vi "slopes2zern.vi"(0 "HasoSlopes in":refnum<class "HasoSlopes.lvclass">, 3 "error in (no error)":errorcluster, 4 "idxType":enum16{"Wyant", "ANSI"}(ring)) -> (6 "HasoSlopes out":refnum<class "HasoSlopes.lvclass">, 7 "Zernike Coefficients":dbl[](graph), 8 "Measured pupil":i32[][](graph), 9 "Zernike pupil":i32[][](graph), 10 "error out":errorcluster)   [LabVIEW 2018]
uses:
  <userlib>/WaveKit.lib/Controls/HasoSlopes.lvclass
  <userlib>/WaveKit.lib/Classes/ComputePhaseSet/ComputePhaseSet.lvclass
  <userlib>/WaveKit.lib/Controls/Pupil.lvclass
  <userlib>/WaveKit.lib/Controls/CircularPupilDetectionParams.ctl
  <userlib>/WaveKit.lib/Controls/PupilDetectionOption.ctl
  <userlib>/WaveKit.lib/Controls/CircularAutoDetectionOptions.ctl
  <userlib>/WaveKit.lib/Controls/PupilDetectionMode.ctl
  <userlib>/WaveKit.lib/Controls/ZernikeModalPrefs.ctl
  <userlib>/WaveKit.lib/Controls/ZernikeProjectionPupilSetup.ctl
  <userlib>/WaveKit.lib/Controls/Point2Df.ctl
  <userlib>/WaveKit.lib/Classes/ModalCoef/ModalCoef.lvclass
  <userlib>/WaveKit.lib/Controls/WavefrontReconstructionMode.ctl
  <userlib>/WaveKit.lib/Controls/WavefrontModalReconstructionType.ctl
  <userlib>/WaveKit.lib/Classes/HasoData/HasoData.lvclass
  <vilib>/Analysis/1siggen.llb/Ramp Pattern by Delta.vi
  <vilib>/Analysis/NI_AALBase.lvlib
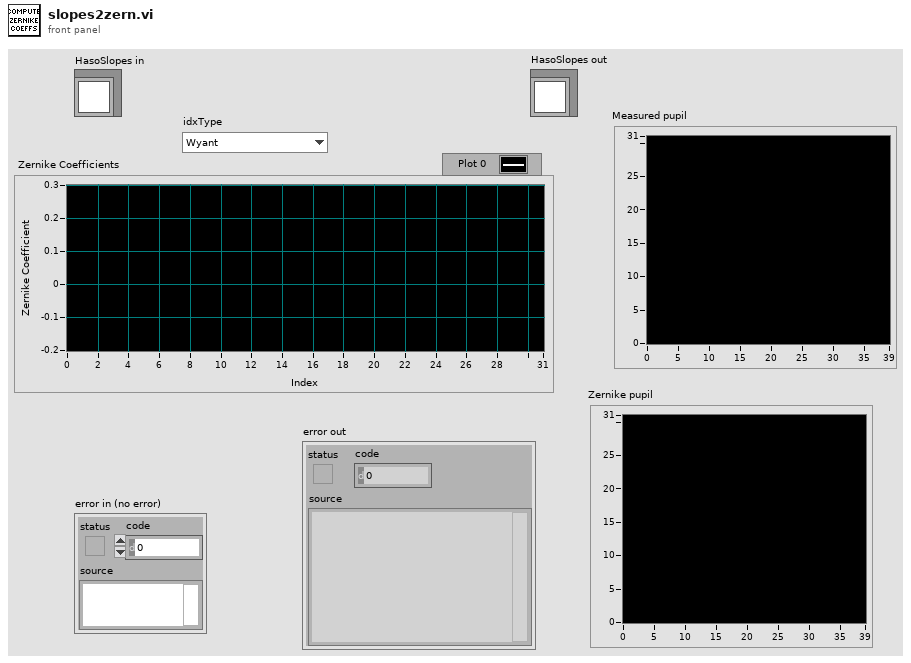
[diagram p1: front panel]
types:
  T1 = typedef "WavefrontModalReconstructionType.ctl" = enum16{"Legendre", "Zernike"}
  T2 = typedef "WavefrontReconstructionMode.ctl" = enum16{"None", "Modal_Legendre", "Modal_Zernike", "Zonal", "Modal_Zonal_Zernike", "Modal_Zonal_Legendre"}
  T3 = typedef "ZernikeModalPrefs.ctl" = cluster{"Number of coefficients":u32, "Filtered coefficients":u32[], "RMS Zernike normalization":bool, "CircularProjectionPupilDimensions":T4}
  T4 = typedef "ZernikeProjectionPupilSetup.ctl" = cluster{"Pupil center_sspp":T5, "Pupil radius_sspp":sgl}
  T5 = typedef "Point2Df.ctl" = cluster{"X":sgl, "Y":sgl}
  T6 = typedef "CircularPupilDetectionParams.ctl" = cluster{"PupilDetectionOption":T7, "AutoDetectionOption":T8, "PupilDetectionMode":T9, "CentralOccultationDetection":bool}
  T7 = typedef "PupilDetectionOption.ctl" = enum16{"Manual", "Automatic"}
  T8 = typedef "CircularAutoDetectionOptions.ctl" = enum16{"manual_radius_auto_center", "manual_center_auto_radius", "auto_radius_auto_center"}
  T9 = typedef "PupilDetectionMode.ctl" = enum16{"inscribed", "circumscribed"}
  T10 = enum16{"ANSI2Wyant", "Wyant2ANSI", "ANSI2ANSI", "Wyant2Wyant"}
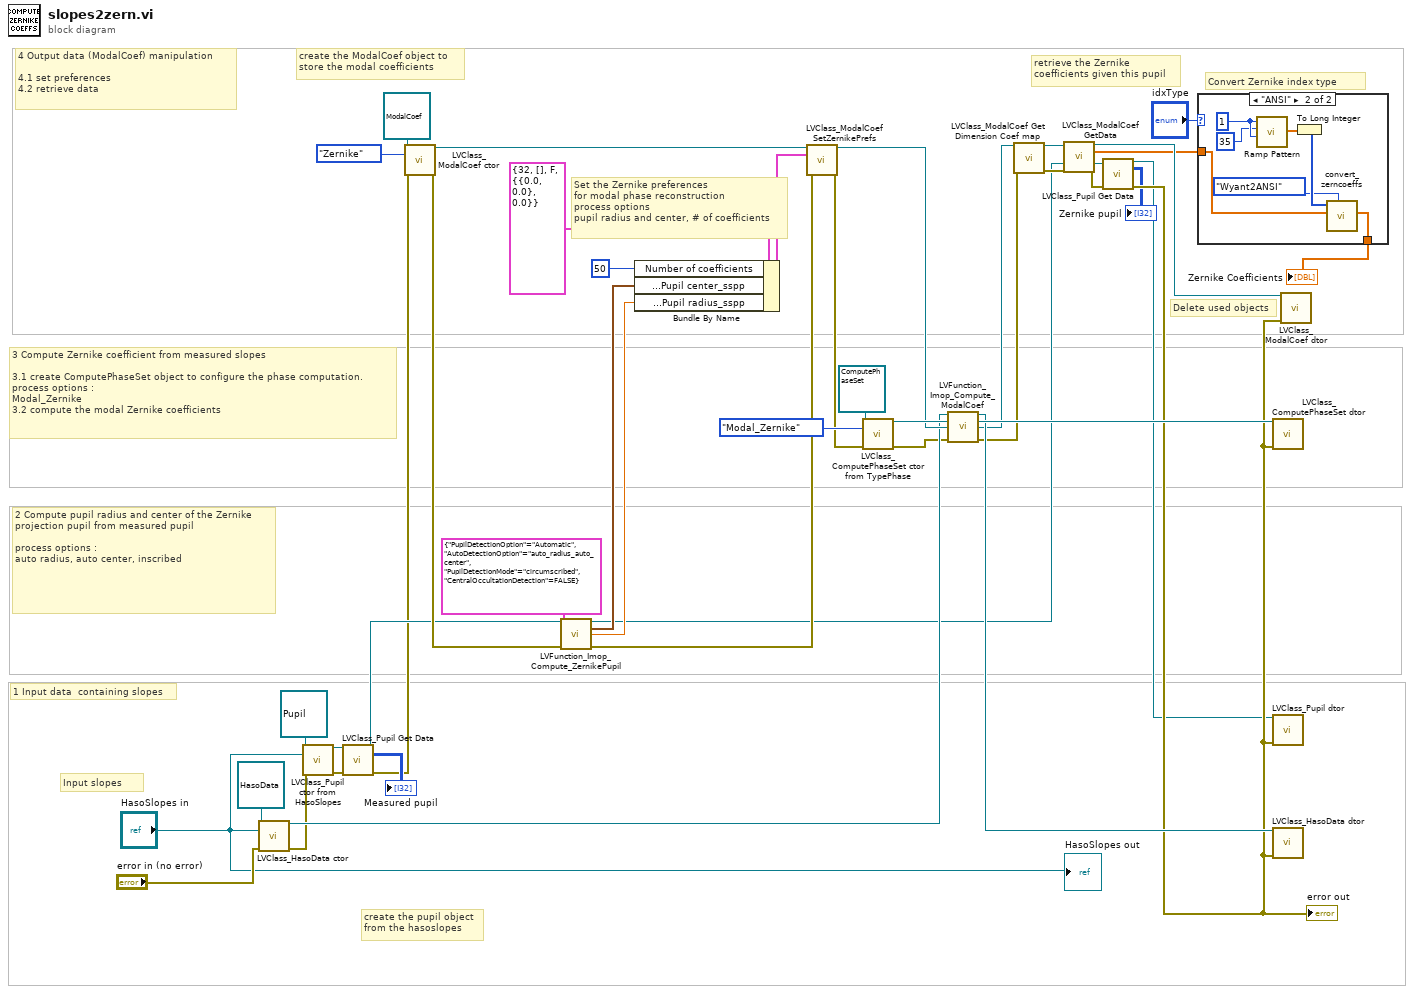
[diagram p0: block diagram]
diagram:
  # "Convert Zernike index type"
  # "Input slopes"
  # "Delete used objects"
  # "4 Output data (ModalCoef) manipulation\n\n4.1 set preferences\n4.2 retrieve data"
  # "retrieve the Zernike\ncoefficients given this pupil"
  # "create the ModalCoef object to\nstore the modal coefficients"
  # "3 Compute Zernike coefficient from measured slopes\n\n3.1 create ComputePhaseSet object to configure the phase computation.\nprocess options :\nModal_Zernike\n3.2 compute the modal Zernike coefficients"
  # "2 Compute pupil radius and center of the Zernike\nprojection pupil from measured pupil\n\nprocess options :\nauto radius, auto center, inscribed"
  # "1 Input data  containing slopes"
  # "Set the Zernike preferences\nfor modal phase reconstruction\nprocess options\npupil radius and center, # of coefficients"
  # "create the pupil object\nfrom the hasoslopes"
  n1 = call <userlib>:"LVClass_HasoData ctor.vi"("HasoData in"=refnum<class "HasoData.lvclass"> refnum, "HasoSlopes.lvclass"="HasoSlopes in", "error in (no error)"="error in (no error)") -> ("HasoData out"=w24:refnum<class "HasoData.lvclass">, "error out"=w22:errorcluster)  [unwired: 11 in]
  n2 = call <userlib>:"LVClass_Pupil ctor from HasoSlopes.vi"("Pupil in"=refnum<class "Pupil.lvclass"> refnum, "HasoSlopes.lvclass"="HasoSlopes in", "error in (no error)"=w22) -> ("Pupil out"=w20:refnum<class "Pupil.lvclass">, "error out"=w18:errorcluster)  [unwired: 11 in]
  n3 = call <userlib>:"LVClass_Pupil Get Data.vi"("Pupil in"=w20, "error in (no error)"=w18) -> ("Pupil out"=w19:refnum<class "Pupil.lvclass">, "Data"=→"Measured pupil":i32[][], "error out"=w8:errorcluster)  [unwired: 11 in]
  n4 = call <userlib>:"LVClass_ModalCoef ctor.vi"("ModalCoef in"=refnum<class "ModalCoef.lvclass"> refnum, "TypePhase"=WavefrontModalReconstructionType."Zernike", "error in (no error)"=w8) -> ("ModalCoef out"=w26:refnum<class "ModalCoef.lvclass">, "error out"=w21:errorcluster)  [unwired: 11 in]
  n5 = call <userlib>:"LVFunction_Imop_Compute_ZernikePupil.vi"("Pupil.lvclass"=w19, "CircularPupilDetectionParams"=T6 {"PupilDetectionOption"=enum."Automatic", "AutoDetectionOption"=enum."auto_radius_auto_center", "PupilDetectionMode"=enum."circumscribed", "CentralOccultationDetection"=FALSE}, "error in"=w21) -> ("Pupil.lvclass"=w15:refnum<class "Pupil.lvclass">, "center"=w32:T5, "radius"=w31:sgl, "error out"=w16:errorcluster)  [unwired: 9 in]
  n6 = Bundle By Name(cluster=T3 {"Number of coefficients"=32, "Filtered coefficients"=[], "RMS Zernike normalization"=FALSE, "CircularProjectionPupilDimensions"={"Pupil center_sspp"={"X"=0.0, "Y"=0.0}, "Pupil radius_sspp"=0.0}} ("ZernikeModalPrefs"), "Number of coefficients"=u32 50, "CircularProjectionPupilDimensions.Pupil center_sspp"=w32, "CircularProjectionPupilDimensions.Pupil radius_sspp"=w31) -> (w33:T3)
  n7 = call <userlib>:"LVClass_ModalCoef SetZernikePrefs.vi"("ModalCoef in"=w26, "ZernikeModalPrefs"=w33, "error in (no error)"=w16) -> ("ModalCoef out"=w27:refnum<class "ModalCoef.lvclass">, "error out"=w7:errorcluster)  [unwired: 11 in]
  n8 = call <userlib>:"LVClass_ComputePhaseSet ctor from TypePhase.vi"("ComputePhaseSet in"=refnum<class "ComputePhaseSet.lvclass"> refnum, "TypePhase"=WavefrontReconstructionMode."Modal_Zernike", "error in (no error)"=w7) -> ("ComputePhaseSet out"=w28:refnum<class "ComputePhaseSet.lvclass">, "error out"=w6:errorcluster)  [unwired: 11 in]
  n9 = call <userlib>:"LVFunction_Imop_Compute_ModalCoef.vi"("HasoData.lvclass"=w24, "ComputePhaseSet.lvclass"=w28, "ModalCoef.lvclass"=w27, "error constant"=w6) -> ("HasoData.lvclass (dup)"=w38:refnum<class "HasoData.lvclass">, "ComputePhaseSet.lvclass (dup)"=w39:refnum<class "ComputePhaseSet.lvclass">, "ModalCoef.lvclass (dup)"=w23:refnum<class "ModalCoef.lvclass">, "error out"=w35:errorcluster)  [unwired: 8 in]
  n10 = call <userlib>:"LVClass_ModalCoef Get Dimension Coef map.vi"("ModalCoef in"=w23, "error in (no error)"=w35) -> ("ModalCoef out"=w40:refnum<class "ModalCoef.lvclass">, "error out"=w36:errorcluster)  [unwired: 11 in, 1 out]
  n11 = call <userlib>:"LVClass_ModalCoef GetData.vi"("ModalCoef in"=w40, "Pupil.lvclass"=w15, "error in (no error)"=w36) -> ("ModalCoef out"=w37:refnum<class "ModalCoef.lvclass">, "coef"=w2:sgl[], "Pupil.lvclass (dup)"=w13:refnum<class "Pupil.lvclass">, "error out"=w12:errorcluster)  [unwired: 8 in, 1 out]
  n12 = call <userlib>:"LVClass_Pupil Get Data.vi"("Pupil in"=w13, "error in (no error)"=w12) -> ("Pupil out"=w10:refnum<class "Pupil.lvclass">, "Data"=→"Zernike pupil":i32[][], "error out"=w11:errorcluster)  [unwired: 11 in]
  "error out" <- w11
  n13 = case shown="\"ANSI\"" "idxType" {
    tunnel: w2 -> [w45 w51]
    tunnel: [w45 w52] -> w1
    frame "Wyant", Default {
    }
    frame "ANSI" {
      w49 = 1
      n14 = call-poly <vilib>:"Ramp Pattern.vi"("start"=w49, "end"=35, "delta"=w49) -> ("Ramp Pattern"=w50:dbl[])  [unwired: 6 in, 2 out]
      n15 = To Long Integer(number=w50) -> (32bit integer=w47:i32[])
      n16 = call "convert_zerncoeffs.vi"("ConType"=T10."Wyant2ANSI", "Zern coef in"=w51, "Zern indx in"=w47) -> ("Zern Coef Out"=w52:dbl[])  [unwired: 6 in, 2 out]
    }
  }
  "Zernike Coefficients" <- w1
  n17 = call <userlib>:"LVClass_ComputePhaseSet dtor.vi"("ComputePhaseSet in"=w39, "error in (no error)"=w11) -> ()  [unwired: 12 in, 2 out]
  n18 = call <userlib>:"LVClass_Pupil dtor.vi"("Pupil in"=w10, "error in (no error)"=w11) -> ()  [unwired: 12 in, 2 out]
  n19 = call <userlib>:"LVClass_HasoData dtor.vi"("HasoData in"=w38, "error in (no error)"=w11) -> ()  [unwired: 12 in, 2 out]
  n20 = call <userlib>:"LVClass_ModalCoef dtor.vi"("ModalCoef in"=w37, "error in (no error)"=w11) -> ()  [unwired: 12 in, 2 out]
  "HasoSlopes out" <- "HasoSlopes in"
